vi "Add Node.vi"(7 "Action (Add)":T1, 8 "error in (no error)":errorcluster, 9 "Node Data":T5, 10 "New Node Path (parent, child)":string[](array[string]), 11 "Tree Map Handle In":T2) -> (0 "error out":errorcluster, 2 "Node Data Replaced?":bool, 3 "Tree Map Handle Out":T2)   [LabVIEW 2020, in "Blue Tree Map OpenSource.lvlib"]
doc: "Add a new node to the tree map.\n\nThere are 2 Action options:\n<B>Add or Modify Node</B> - This will create a new node if the node is not found. This will happen recursively, which means that multiple new nodes might be created. If the node already exists, then the node data will be replaced.\n<B>Modify Node only if found</B> - This will replace the node data if the node path is found. Otherwise, nothing happens.\n\nThe New Node Path input is not allowed to contain any characters specific in the tree map \"delimiter.\" This function will stop recursing when an invalid path name is found."
uses:
  Blue Tree Map OpenSource.lvlib
  Typedefs/Tree Node Data.ctl
  Typedefs/Attribute Map.ctl
  Typedefs/Tree Map Handle.ctl
  Typedefs/Tree Map.ctl
  Typedefs/Tree Map Data.ctl
  Typedefs/AddNodeAction.ctl
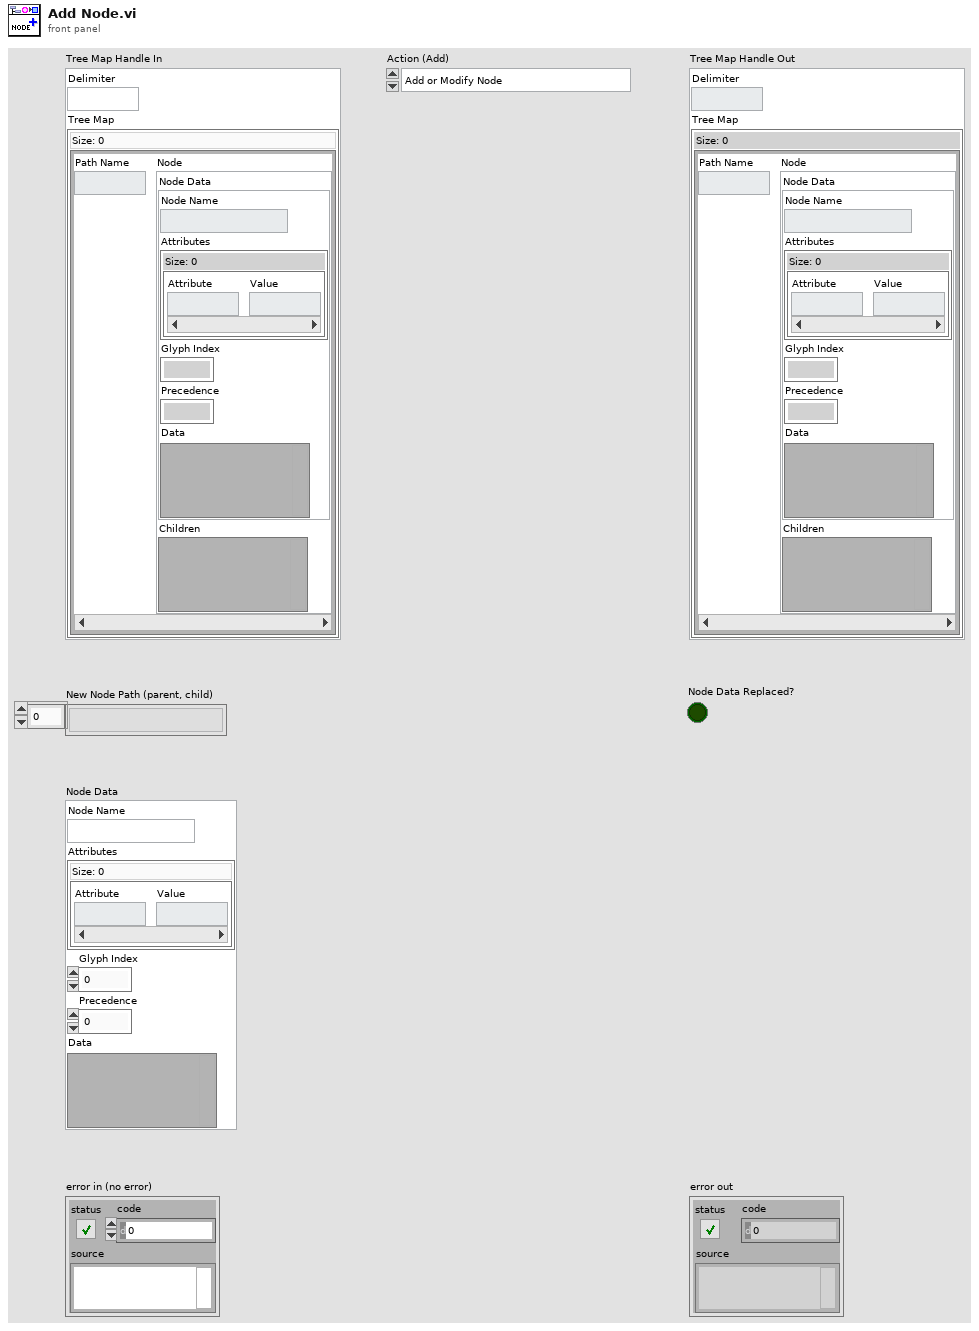
[diagram p1: front panel]
types:
  T1 = typedef "Blue Tree Map OpenSource.lvlib/AddNodeAction.ctl" = enum16{"Add or Modify Node", "Modify Node only if found"}
  T2 = typedef "Blue Tree Map OpenSource.lvlib/Tree Map Handle.ctl" = cluster{"Delimiter":string, "Tree Map":T3}
  T3 = typedef "Blue Tree Map OpenSource.lvlib/Tree Map.ctl" = map{string, T4}
  T4 = typedef "Blue Tree Map OpenSource.lvlib/Tree Map Data.ctl" = cluster{"Node Data":T5, "Children":variant}
  T5 = typedef "Blue Tree Map OpenSource.lvlib/Tree Node Data.ctl" = cluster{"Node Name":string, "Attributes":T6, "Glyph Index":i32, "Precedence":i32, "Data":variant}
  T6 = typedef "Blue Tree Map OpenSource.lvlib/Attribute Map.ctl" = map{string, string}
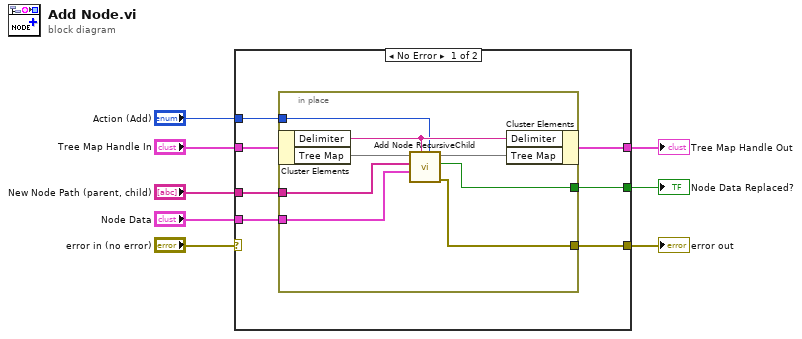
[diagram p0: block diagram]
diagram:
  n1 = case shown="No Error" "error in (no error)" {
    selector: "error in (no error)" -> [_ w25]
    tunnel: "New Node Path (parent, child)" -> [w15 _]
    tunnel: [w14 w25] -> w6
    tunnel: [w13 _] -> w5
    tunnel: "Node Data" -> [w12 _]
    tunnel: "Tree Map Handle In" -> [w11 w24]
    tunnel: [w10 w24] -> w2
    tunnel: "Action (Add)" -> [w9 _]
    frame No Error {
      n2 = in-place {
        in-place-border: w15 -> [w20]
        in-place-border: [w17] -> w14
        in-place-border: [w18] -> w13
        in-place-border: w12 -> [w19]
        in-place-border: w9 -> [w16]
        n3 = in-place-cluster #1(w11) -> ("Delimiter"=w22:string, "Tree Map"=w23:T3)
        n4 = call "Add Node RecursiveChild.vi"("Action"=w16, "Delimiter"=w22, "Node Data"=w19, "New Node Path (parent, child)"=w20, "Tree Map In"=w23) -> ("error out"=w17:errorcluster, "Node Data Replaced?"=w18:bool, "Tree Map Out"=w21:T3)  [unwired: 4 in]
        n5 = in-place-cluster #1("Delimiter"=w22, "Tree Map"=w21) -> (w10:T2)
      }
    }
    frame Error {
    }
  }
  "error out" <- w6
  "Node Data Replaced?" <- w5
  "Tree Map Handle Out" <- w2
